vi "path steer3.vi"(11 "lane":bool) -> (2 "curve vel limit":dbl, 3 "handle":dbl=175.61695170488764)   [LabVIEW 2015]
uses:
  <vilib>/Analysis/7linalg.llb/Solve Linear Equations (single right hand).vi
  <vilib>/Analysis/baseanly.llb/Solve Linear Equations By Cholesky.vi
  <vilib>/Analysis/baseanly.llb/Real Matrix to Compact Array.vi
  <vilib>/Analysis/baseanly.llb/Real Compact Tri-Matrix Linear Eqs.vi
  G_ALL.vi
  <vilib>/Analysis/7linalg.llb/Solve Linear Eqs (General).vi
  <vilib>/Analysis/7linalg.llb/Solve Linear Eqs (Gen, single right hand).vi
  <vilib>/Analysis/NI_AALPro.lvlib
panel:
  out "path end":bool
  in  "an[g]":dbl=-0.17 format="%#_13g"
  out "Waveform Graph":dynamicdata(graph)
  in  "mu":dbl=0.005 format="%#_13g"
  in  "dx gain":dbl=0.019999999999999997 min=0.0 max=0.2 step=0.01
  out "x value":dbl=-0.8542483758567541
  out "XY Graph":cluster{"Y":dbl[], "Y":dbl[]}[](graph)=[{"Y"=[-5.246809304707959, -4.763210909809536, -4.298248751776158, -3.853163667485589, -3.4268765479315446, -3.029477672753705, -2.6673284986480974, -2.335336691519628, -2.0366453167866156, -1.7750835921098853, -1.5528767688369498, -1.3644656447475765, -1.2079630605299954, -1.074690008661569, -0.9585132340675446, -0.8551782329420596, -0.7665829934540727, -0.6868993462607671, -0.6126823280970868, -0.5442164343365972, -0.47614894814750475, -0.41410047141640827, -0.3538150238541624, -0.29540366128691464, -0.24219086500490516, -0.19691528446819184, -0.15547027846011519, -0.11340295527325328, -0.07144915398020535, -0.03434793001665748, 0.0, 0.026526158792223087, 0.05124494389382517, 0.07270742281515652, 0.06435385726912624, -0.004553363938687882, -0.139882839282637, -0.3359547912247316, -0.5900103181212502, -0.900040761768828, -1.2577413584671457, -1.66216965308078, -2.1012210225275174, -2.5653232377446606, -3.0450206197370466, -3.5404770109177743, -4.039369871326692, -4.541851143281866, -5.046387603513992, -5.553897537492966, -6.061637927692216, -6.567645563226444, -7.068648217182836, -7.570715384980373, -8.064438697718192, -8.545111556606587, -8.998477174205098, -9.422019565773061, -9.805695724849244, -10.146105279341642], "Y"=[-13.12635530502614, -12.964543503689939, -12.76763447744193, -12.524937360608902, -12.2475735581719, -11.933583222485607, -11.583671941038977, -11.206464906204559, -10.79245190322264, -10.354599285401152, -9.898639757724679, -9.426030687571156, -8.945680321385996, -8.454465203163156, -7.963985068856038, -7.468786738899853, -6.97312085053041, -6.479311060157665, -5.971731167568438, -5.469535412616666, -4.9636888467403155, -4.464752828537232, -3.9649913085777393, -3.458342585235778, -2.9601418499725303, -2.459972000641257, -1.9586644185731306, -1.4494467342092758, -0.9454480119816643, -0.4403687170997531, 0.06136222931732077, 0.5678735764406926, 1.068808881478275, 1.5686590067794068, 2.0720530905057277, 2.5736288544042853, 3.0594879994083963, 3.5248827445502124, 3.9579216058298154, 4.3560080630331335, 4.707794061133773, 5.011781058067703, 5.259264085768475, 5.451142759582283, 5.593309208559008, 5.693936293621469, 5.758617125078806, 5.791664966026638, 5.794000380643315, 5.784136801290129, 5.782533687658117, 5.785062966223215, 5.79993550563809, 5.8290421589798, 5.9156579447766475, 6.067163605595132, 6.278887512503447, 6.54911596168099, 6.871713294872911, 7.24413426029683]}, {"Y"=[-27.79054311036769, -27.788426793206575, -27.782078486373944, -27.77150012362555, -27.75669492723317, -27.737667407003034, -27.71442335890214, -27.686969863292695, -27.655315282775426, -27.619469259642194, -27.5794427129389, -27.5352478351394, -27.48689808843162, -27.434408200616765, -27.377794160623147, -27.317073213635787, -27.25226385584335, -27.18338582880404, -27.110460113432133, -27.033508923606977, -26.95255569940644, -26.867625099966816, -26.77874299597144, -26.68593646177021, -26.589233767132484, -26.488664368635824, -26.384258900693254, -26.2760491662217, -26.16406812695454, -26.048349893401117, -25.92892971445636, -25.805843966663623, -25.679130143134046, -25.548826842125777, -25.41497375528658, -25.27761165556337, -25.13678238478238, -24.992528840903734, -24.844894964954314, -24.693925727642892, -24.53966711566163, -24.382166117678068, -24.221470710021944, -24.057629842071115, -23.890693421341133, -23.720712298282884, -23.547738250793113, -23.37182396844231, -23.193023036425007, -23.011389919237175, -22.82697994408583, -22.639849284035826, -22.450054940898987, -22.257654727870808, -22.062707251920006, -21.865271895936253, -21.66540880064158, -21.463178846270928, -21.25864363402745, -21.05186546731817, -20.84290733277577, -20.631832881072256, -20.41870640753034, -20.20359283253847, -19.986557681775434, -19.767667066250628, -19.54698766216598, -19.324586690605734, -19.10053189706029, -18.874891530790215, -18.64773432403691, -18.419129471086073, -18.18914660719046, -17.957855787358298, -17.725327465013883, -17.491632470536747, -17.256841989686063, -17.02102754191677, -16.784260958594032, -16.546614361112756, -16.308160138928653, -16.068970927507767, -15.829119586200973, -15.588679176050324, -15.347722937533948, -15.106324268256303, -14.864556700590517, -14.622493879279771, -14.38020953900434, -14.137777481921338, -13.895271555183845, -13.652765628446353, -13.410333571363354, -13.16804923108792, -12.92598640977717, -12.684218842111388, -12.442820172833741, -12.20186393431737, -11.961423524166722, -11.721572182859921, -11.482382971439037, -11.243928749254936, -11.006282151773657, -10.769515568450924, -10.533701120681629, -10.298910639830943, -10.06521564535381, -9.832687323009392, -9.601396503177233, -9.37141363928162, -9.142808786330779, -8.915651579577474, -8.690011213307402, -8.465956419761957, -8.243555448201716, -8.022876044117066, -7.803985428592254, -7.586950277829223, -7.371836702837354, -7.158710229295436, -6.947635777591925, -6.738677643049522, -6.531899476340242, -6.32736426409676, -6.125134309726112, -5.925271214431441, -5.727835858447683, -5.53288838249688, -5.3404881694687045, -5.150693826331867, -4.96356316628186, -4.779153191130517, -4.597520073942688, -4.418719141925381, -4.242804859574576, -4.069830812084804, -3.8998496890265617, -3.7329132682965724, -3.5690724003457444, -3.4083769926896217, -3.250875994706062, -3.096617382724796, -2.9456481454133776, -2.798014269463957, -2.6537607255853093, -2.5129314548043187, -2.3755693550811117, -2.241716268241916, -2.1114129672336457, -1.9846991437040682, -1.8616133959113306, -1.7421932169665748, -1.62647498341315, -1.5144939441459915, -1.406284209674439, -1.3018787417318656, -1.201309343235204, -1.1046066485974766, -1.0118001143962498, -0.9229180104008776, -0.8379874109612526, -0.7570341867607127, -0.6800829969355568, -0.6071572815636515, -0.5382792545243404, -0.47346989673190265, -0.41274894974454135, -0.3561349097509261, -0.30364502193607024, -0.25529527522828666, -0.21110039742879394, -0.1710738507254952, -0.13522782759226182, -0.10357324707499238, -0.07611975146555316, -0.052875703364655635, -0.03384818313452165, -0.019042986742137558, -0.00846462399374559, -0.0021163171611142673, 0.0, -0.0021163171611142673, -0.00846462399374559, -0.019042986742137558, -0.03384818313452165, -0.052875703364655635, -0.07611975146555316, -0.10357324707499238, -0.13522782759226182, -0.17107385072549341, -0.21110039742879394, -0.25529527522828666, -0.30364502193607024, -0.3561349097509261, -0.4127489497445396, -0.4734698967319009, -0.5382792545243387, -0.6071572815636497, -0.6800829969355586, -0.7570341867607127, -0.8379874109612526, -0.9229180104008758, -1.011800114396248, -1.1046066485974766, -1.2013093432352022, -1.3018787417318638, -1.4062842096744355, -1.5144939441459861, -1.6264749834131482, -1.7421932169665766, -1.8616133959113323, -1.9846991437040664, -2.111412967233644, -2.2417162682419143, -2.37556935508111, -2.512931454804317, -2.6537607255853075, -2.798014269463952, -2.9456481454133705, -3.0966173827247943, -3.2508759947060604, -3.4083769926896235, -3.569072400345746, -3.7329132682965707, -3.89984968902656, -4.069830812084803, -4.242804859574575, -4.418719141925379, -4.597520073942681, -4.77915319113051, -4.9635631662818565, -5.150693826331869, -5.340488169468708, -5.532888382496882, -5.727835858447682, -5.925271214431433, -6.125134309726104, -6.3273642640967624, -6.531899476340239, -6.738677643049519, -6.947635777591917, -7.158710229295428, -7.371836702837351, -7.58695027782922, -7.803985428592251, -8.022876044117067, -8.243555448201715, -8.465956419761955, -8.6900112133074, -8.915651579577467, -9.14280878633077, -9.371413639281617, -9.601396503177229, -9.832687323009386, -10.065215645353812, -10.298910639830945, -10.533701120681625, -10.769515568450919, -11.006282151773648, -11.24392874925494, -11.482382971439037, -11.721572182859921, -11.961423524166714, -12.201863934317359, -12.442820172833729, -12.684218842111388, -12.925986409777169, -13.168049231087927, -13.410333571363354, -13.652765628446351, -13.895271555183843, -14.137777481921333, -14.380209539004332, -14.622493879279759, -14.864556700590516, -15.106324268256296, -15.347722937533955, -15.588679176050325, -15.82911958620097, -16.068970927507763, -16.30816013892865, -16.546614361112745, -16.784260958594036, -17.021027541916766, -17.25684198968606, -17.49163247053674, -17.725327465013873, -17.957855787358298, -18.189146607190455, -18.41912947108607, -18.647734324036914, -18.874891530790215, -19.100531897060286, -19.32458669060573, -19.546987662165968, -19.767667066250617, -19.986557681775434, -20.203592832538465, -20.418706407530333, -20.631832881072256, -20.842907332775766, -21.051865467318166, -21.258643634027447, -21.46317884627092, -21.66540880064158, -21.865271895936253, -22.062707251920003, -22.257654727870804, -22.45005494089898, -22.63984928403582, -22.826979944085828, -23.01138991923717, -23.19302303642501, -23.371823968442314, -23.54773825079311, -23.720712298282884, -23.890693421341126, -24.057629842071112, -24.221470710021936, -24.382166117678068, -24.539667115661626, -24.693925727642895, -24.844894964954314, -24.992528840903734, -25.13678238478238, -25.277611655563366, -25.414973755286574, -25.548826842125777, -25.679130143134046, -25.805843966663623, -25.928929714456356, -26.04834989340111, -26.16406812695454, -26.276049166221696, -26.384258900693247, -26.488664368635824, -26.589233767132484, -26.68593646177021, -26.778742995971438, -26.867625099966812, -26.95255569940643, -27.033508923606977, -27.110460113432133, -27.183385828804038, -27.25226385584335, -27.317073213635787, -27.377794160623147, -27.434408200616765, -27.486898088431616, -27.535247835139405, -27.5794427129389, -27.619469259642194, -27.655315282775426, -27.686969863292695, -27.71442335890214, -27.737667407003034, -27.75669492723317, -27.77150012362555, -27.782078486373944, -27.788426793206575], "Y"=[-0.0, -0.24250592673749302, -0.48493798382049413, -0.7272223240959237, -0.969285145406673, -1.2110527130724553, -1.4524513823501046, -1.6934076208664777, -1.9338480310171269, -2.1736993723239215, -2.4128885837448077, -2.6513428059289086, -2.8889894034101893, -3.1257559867329223, -3.3615704345022186, -3.596360915352901, -3.830055909830037, -4.062584232174453, -4.293875052006613, -4.52385791590223, -4.752462768853066, -4.97961997560637, -5.205260341876442, -5.429315135421889, -5.65171610698213, -5.872395511066782, -6.091286126591589, -6.308321277354623, -6.523434852346495, -6.736561325888409, -6.9476357775919215, -7.156593912134322, -7.363372078843605, -7.567907291087082, -7.770137245457733, -7.970000340752407, -8.167435696736161, -8.362383172686963, -8.55478338571514, -8.744577728851981, -8.931708388901985, -9.11611836405333, -9.29775148124116, -9.476552413258466, -9.652466695609267, -9.82544074309904, -9.995421866157285, -10.162358286887272, -10.326199154838099, -10.486894562494223, -10.644395560477784, -10.798654172459047, -10.949623409770469, -11.09725728571989, -11.241510829598536, -11.382340100379524, -11.519702200102733, -11.65355528694193, -11.783858587950201, -11.910572411479777, -12.033658159272512, -12.15307833821727, -12.268796571770693, -12.380777611037853, -12.488987345509406, -12.59339281345198, -12.693962211948639, -12.790664906586368, -12.883471440787595, -12.97235354478297, -13.057284144222592, -13.138237368423132, -13.215188558248288, -13.288114273620195, -13.356992300659504, -13.421801658451942, -13.482522605439303, -13.539136645432919, -13.591626533247775, -13.639976279955558, -13.684171157755053, -13.72419770445835, -13.760043727591583, -13.791698308108852, -13.819151803718292, -13.84239585181919, -13.861423372049323, -13.876228568441707, -13.8868069311901, -13.89315523802273, -13.895271555183845, -13.89315523802273, -13.8868069311901, -13.876228568441707, -13.861423372049323, -13.84239585181919, -13.819151803718293, -13.791698308108852, -13.760043727591583, -13.72419770445835, -13.684171157755053, -13.639976279955558, -13.591626533247775, -13.53913664543292, -13.482522605439303, -13.421801658451942, -13.356992300659504, -13.288114273620195, -13.215188558248288, -13.138237368423134, -13.057284144222592, -12.972353544782969, -12.883471440787595, -12.790664906586368, -12.69396221194864, -12.593392813451981, -12.488987345509406, -12.380777611037855, -12.268796571770697, -12.153078338217272, -12.033658159272516, -11.910572411479778, -11.783858587950201, -11.65355528694193, -11.519702200102735, -11.382340100379528, -11.241510829598536, -11.09725728571989, -10.949623409770469, -10.79865417245905, -10.644395560477784, -10.486894562494225, -10.326199154838102, -10.162358286887274, -9.995421866157285, -9.825440743099042, -9.65246669560927, -9.476552413258466, -9.297751481241159, -9.11611836405333, -8.931708388901988, -8.74457772885198, -8.554783385715142, -8.362383172686968, -8.167435696736163, -7.9700003407524065, -7.770137245457734, -7.567907291087087, -7.363372078843605, -7.1565939121343245, -6.9476357775919215, -6.7365613258884105, -6.523434852346494, -6.308321277354625, -6.091286126591593, -5.872395511066783, -5.6517161069821285, -5.42931513542189, -5.205260341876445, -4.979619975606376, -4.752462768853069, -4.523857915902228, -4.293875052006615, -4.062584232174458, -3.8300559098300377, -3.596360915352905, -3.361570434502219, -3.1257559867329254, -2.888989403410189, -2.6513428059289113, -2.4128885837448126, -2.1736993723239233, -1.933848031017125, -1.6934076208664786, -1.4524513823501084, -1.2110527130724555, -0.969285145406676, -0.7272223240959296, -0.4849379838204965, -0.24250592673749197, -1.7016237834565482e-15, 0.24250592673748858, 0.4849379838204931, 0.72722232409592, 0.9692851454066664, 1.2110527130724522, 1.4524513823501048, 1.6934076208664814, 1.9338480310171278, 2.1736993723239197, 2.4128885837448095, 2.6513428059289077, 2.8889894034101857, 3.1257559867329223, 3.3615704345022155, 3.5963609153528955, 3.830055909830029, 4.062584232174455, 4.293875052006618, 4.523857915902231, 4.752462768853065, 4.979619975606372, 5.205260341876442, 5.429315135421887, 5.651716106982125, 5.872395511066779, 6.0912861265915845, 6.308321277354616, 6.52343485234649, 6.736561325888413, 6.947635777591924, 7.156593912134322, 7.363372078843602, 7.567907291087084, 7.7701372454577315, 7.970000340752404, 8.16743569673616, 8.36238317268696, 8.554783385715135, 8.744577728851977, 8.931708388901985, 9.116118364053332, 9.29775148124116, 9.476552413258464, 9.652466695609267, 9.825440743099039, 9.995421866157281, 10.162358286887272, 10.326199154838095, 10.48689456249422, 10.644395560477783, 10.798654172459052, 10.94962340977047, 11.09725728571989, 11.241510829598534, 11.382340100379523, 11.51970220010273, 11.653555286941932, 11.7838585879502, 11.910572411479777, 12.03365815927251, 12.153078338217266, 12.268796571770695, 12.380777611037853, 12.488987345509404, 12.593392813451981, 12.69396221194864, 12.790664906586366, 12.883471440787595, 12.972353544782967, 13.057284144222589, 13.138237368423132, 13.215188558248288, 13.288114273620193, 13.356992300659506, 13.421801658451942, 13.482522605439303, 13.539136645432919, 13.591626533247773, 13.63997627995556, 13.684171157755053, 13.72419770445835, 13.760043727591581, 13.791698308108852, 13.819151803718292, 13.84239585181919, 13.861423372049323, 13.876228568441707, 13.8868069311901, 13.89315523802273, 13.895271555183845, 13.89315523802273, 13.8868069311901, 13.876228568441707, 13.861423372049323, 13.84239585181919, 13.819151803718292, 13.791698308108852, 13.760043727591583, 13.724197704458351, 13.684171157755053, 13.63997627995556, 13.591626533247773, 13.539136645432919, 13.482522605439305, 13.421801658451944, 13.356992300659506, 13.288114273620195, 13.21518855824829, 13.138237368423134, 13.05728414422259, 12.972353544782969, 12.883471440787597, 12.79066490658637, 12.693962211948643, 12.593392813451985, 12.488987345509408, 12.380777611037855, 12.268796571770697, 12.15307833821727, 12.033658159272512, 11.910572411479778, 11.783858587950203, 11.653555286941934, 11.519702200102733, 11.382340100379524, 11.241510829598537, 11.097257285719893, 10.949623409770474, 10.798654172459056, 10.644395560477784, 10.486894562494227, 10.326199154838095, 10.16235828688727, 9.995421866157285, 9.825440743099042, 9.65246669560927, 9.47655241325847, 9.29775148124117, 9.11611836405333, 8.931708388901988, 8.744577728851976, 8.554783385715139, 8.362383172686963, 8.167435696736165, 7.970000340752413, 7.770137245457741, 7.567907291087083, 7.363372078843606, 7.156593912134326, 6.947635777591929, 6.736561325888418, 6.523434852346495, 6.308321277354626, 6.091286126591594, 5.872395511066778, 5.65171610698213, 5.429315135421891, 5.205260341876446, 4.979619975606377, 4.752462768853076, 4.52385791590223, 4.293875052006616, 4.062584232174459, 3.8300559098300337, 3.5963609153529004, 3.3615704345022204, 3.125755986732927, 2.888989403410197, 2.651342805928907, 2.4128885837448086, 2.173699372323925, 1.9338480310171329, 1.6934076208664863, 1.4524513823501162, 1.2110527130724573, 0.9692851454066778, 0.7272223240959189, 0.484937983820492, 0.24250592673749366]}]
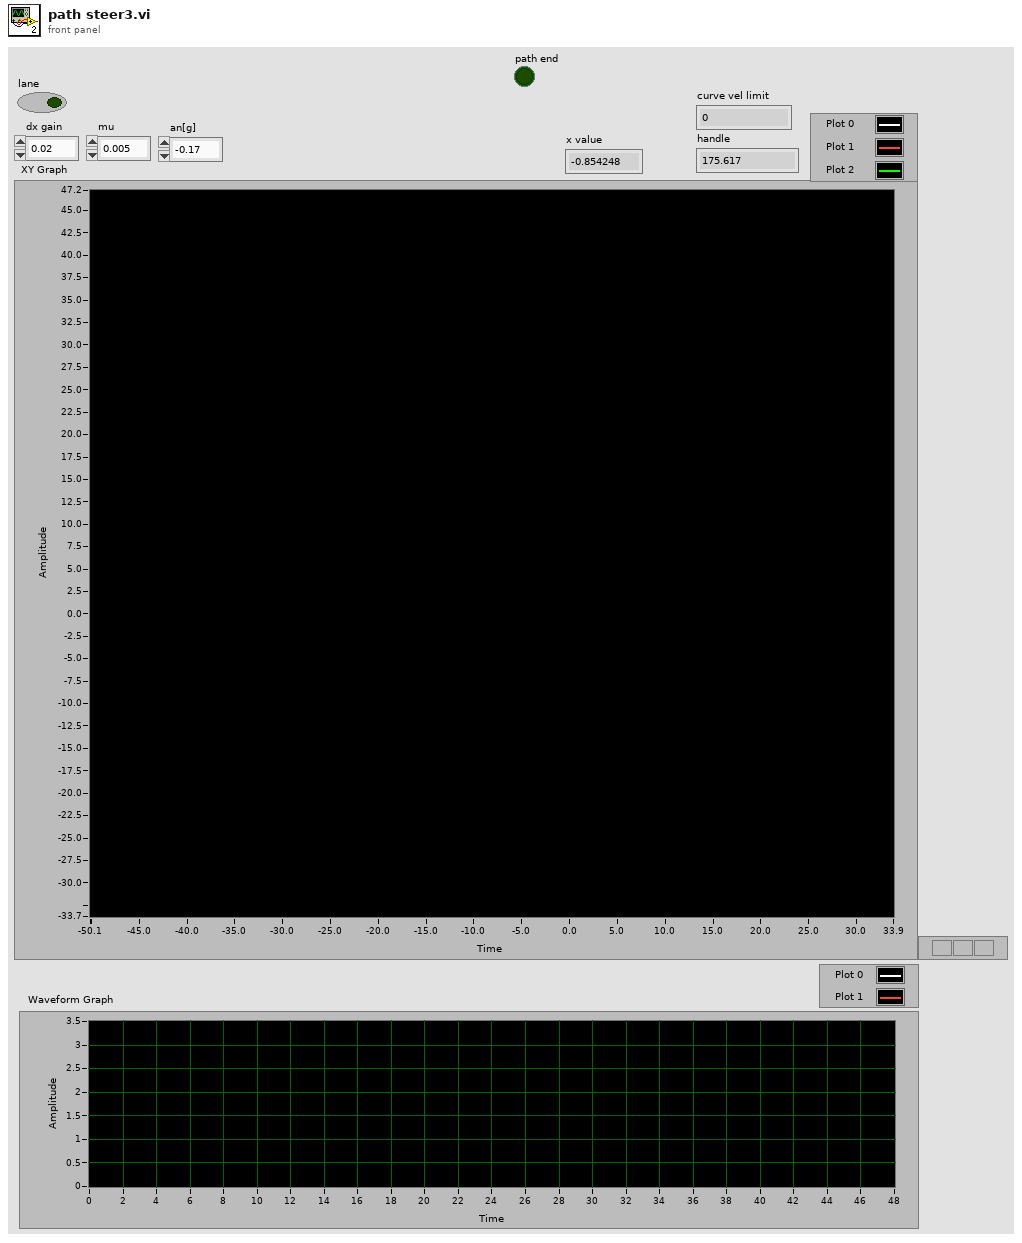
[diagram p1: front panel]
types:
  T1 = cluster{"Steer_input":dbl, "Steer_output":dbl, "VS_des":dbl, "VS_can":dbl, "heading":dbl, "auto":bool, "run":bool, "x":dbl, "y":dbl}
  T2 = cluster{"C_Wheel base":dbl, "ratio_steer":dbl, "Overall width":dbl, "af":dbl, "turn radius":dbl, "eval":dbl, "ap":dbl, "an":dbl, "Vmax":dbl, "mu":dbl, "Vlast":dbl}
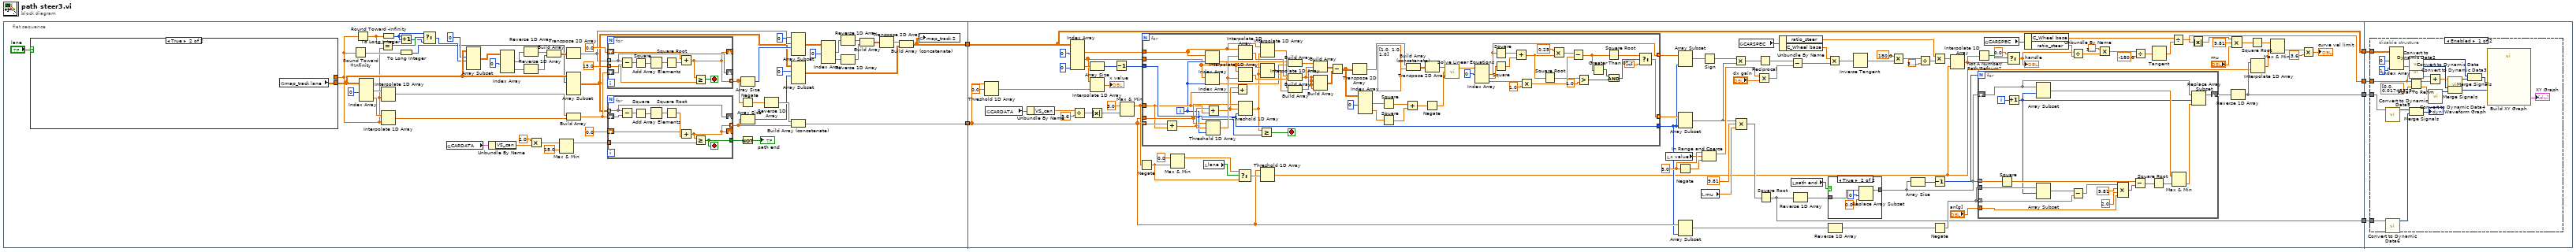
[diagram p0: block diagram]
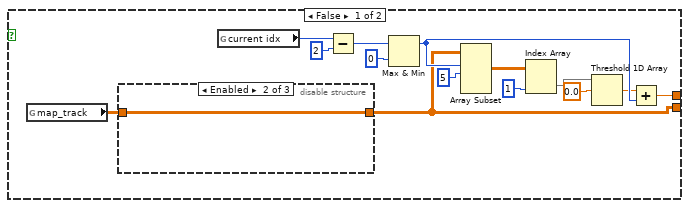
[diagram p2: hidden frame]
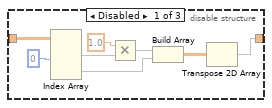
[diagram p3: hidden frame]
diagram:
  n1 = flat-sequence {
    tunnel: [w15] -> w5
    tunnel: [w14] -> w3
    tunnel: [w132] -> w6
    tunnel: w5 -> [w168]
    tunnel: [w168] -> w4
    tunnel: w3 -> [w124]
    tunnel: [w116] -> w2
    tunnel: [w115] -> w1
    tunnel: w6 -> [w276]
    tunnel: w4 -> [w277]
    tunnel: w2 -> [w275]
    tunnel: w1 -> [w274]
    frame #0 {
      n2 = case shown="True" "lane" {
        tunnel: [w63 w86] -> w53
        tunnel: [w65 _] -> w16
        frame False {
          n3 = global read "G_ALL.vi" "map_track"() -> (w64:dbl[][])
          n4 = disable-structure shown="Enabled" {
            disable-tunnel: w64 -> [w84 w85 _]
            disable-tunnel: [w77 w85 _] -> w63
            frame Disabled {
              n5 = Index Array(array=w84, index (col) #1=0 ("disabled index (col)")) -> (element #1=w82:dbl[], element #2=w79:dbl[])  [unwired: 3 in]
              n6 = Multiply(x=1.0, y=w82) -> (x*y=w80:dbl[])
              n7 = Build Array(w80, w79) -> (w78:dbl[][])
              n8 = Transpose 2D Array(2D array=w78) -> (transposed array=w77:dbl[][])
            }
            frame Enabled {
            }
            frame Disabled {
            }
          }
          n9 = global read "G_ALL.vi" "current idx"() -> (w66:i32)
          n10 = Subtract(x=w66, y=2) -> (x-y=w75:i32)
          n11 = Max & Min(x=w75, y=0) -> (max(x,y)=w69:i32)  [unwired: 1 out]
          n12 = Array Subset(array=w63, index (row)=w69, length (row)=5 ("length")) -> (w72:dbl[][])  [unwired: 2 in]
          n13 = Index Array(array=w72, index (col)=1 ("disabled index (col)")) -> (element=w70:dbl[])  [unwired: 1 in]
          n14 = Threshold 1D Array(2:0.0 ("threshold y"), 3:w70) -> (0:w67:dbl)  [unwired: 1 in]
          n15 = Add(x=w67, y=w69) -> (x+y=w65:dbl)
        }
        frame True {
          n16 = global read "G_ALL.vi" "map_track lane"() -> (w86:dbl[][])
        }
      }
      n17 = Round Toward +Infinity(x=w16) -> (ceil(x): smallest int >= x=w24:dbl)
      n18 = Round Toward -Infinity(1:w16) -> (0:w23:dbl)
      n19 = Index Array(array=w53, index (col) #1=0 ("disabled index (col)")) -> (element #1=w61:dbl[], element #2=w60:dbl[])  [unwired: 3 in]
      n20 = Equal?(x=w23, y=w16) -> (x = y?=w22:bool)
      n21 = To Long Integer(number=w23) -> (32bit integer=w20:i32)
      n22 = Interpolate 1D Array(1:w16, 2:w61) -> (0:w59:dbl)
      n23 = Interpolate 1D Array(1:w16, 2:w60) -> (0:w58:dbl)
      n24 = Increment(x=w20) -> (x+1=w19:i32)
      n25 = To Long Integer(number=w24) -> (32bit integer=w18:i32)
      n26 = Select(t=w20, s=w22, f=w19) -> (s? t:f=w21:i32)
      n27 = global read "G_ALL.vi" "CARDATA"() -> (w55:T1)
      n28 = Array Subset(array=w53, index (row)=0 ("index"), length (row)=w21) -> (w51:dbl[][])  [unwired: 2 in]
      n29 = Unbundle By Name(w55) -> ("VS_can"=w13:dbl)
      n30 = Index Array(array=w51, index (col) #1=0 ("disabled index (col)")) -> (element #1=w49:dbl[], element #2=w48:dbl[])  [unwired: 3 in]
      n31 = Reverse 1D Array(array=w49) -> (reversed array=w47:dbl[])
      n32 = Reverse 1D Array(array=w48) -> (reversed array=w46:dbl[])
      n33 = Multiply(x=2.0, y=w13) -> (x*y=w12:dbl)
      n34 = Build Array(w47, w46) -> (w26:dbl[][])
      n35 = Max & Min(x=w12, y=15.0) -> (max(x,y)=w54:dbl)  [unwired: 1 out]
      n36 = Transpose 2D Array(2D array=w26) -> (transposed array=w25:dbl[][])
      n37 = Array Subset(array=w53, index (row)=w18) -> (w28:dbl[][])  [unwired: 3 in]
      n38 = Build Array(w59, w58) -> (w44:dbl[])
      n39 = for {
        tunnel: w25 -> [w89] mode=indexing
        shift-right: [w89] -> _
        shift-left: w44 -> [w96]
        shift-right: [w88] -> _
        shift-left: 0.0 -> [w91]
        tunnel: 15.0 ("y") -> [w90]
        tunnel: [w88] -> w40 mode=indexing
        stop <- w87 stop-if-true
        n40 = Subtract(x=w89, y=w96) -> (x-y=w95:dbl[])
        n41 = Square(x=w95) -> (x^2=w94:dbl[])
        n42 = Add Array Elements(numeric array=w94) -> (sum=w93:dbl)
        n43 = Square Root(x=w93) -> (sqrt(x)=w92:dbl)
        n44 = Add(x=w91, y=w92) -> (x+y=w88:dbl)
        n45 = Greater Or Equal?(x=w88, y=w90) -> (x >= y?=w87:bool)
      }
      n46 = for {
        tunnel: w28 -> [w99] mode=indexing
        shift-right: [w99] -> _
        shift-left: w44 -> [w106]
        shift-right: [w98] -> _
        shift-left: 0.0 -> [w101]
        tunnel: w54 -> [w100]
        tunnel: [w98] -> w27 mode=indexing
        tunnel: [w97] -> w8
        stop <- w97 stop-if-true
        n47 = Subtract(x=w99, y=w106) -> (x-y=w105:dbl[])
        n48 = Square(x=w105) -> (x^2=w104:dbl[])
        n49 = Add Array Elements(numeric array=w104) -> (sum=w103:dbl)
        n50 = Square Root(x=w103) -> (sqrt(x)=w102:dbl)
        n51 = Add(x=w101, y=w102) -> (x+y=w98:dbl)
        n52 = Greater Or Equal?(x=w98, y=w100) -> (x >= y?=w97:bool)
      }
      n53 = Negate(x=w40) -> (-x=w42:dbl[])
      n54 = Not(x=w8) -> (.not. x?=→"path end":bool)
      n55 = Array Size(array=w40) -> (size(s)=w38:i32)
      n56 = Array Size(array=w27) -> (size(s)=w9:i32)
      n57 = Reverse 1D Array(array=w42) -> (reversed array=w41:dbl[])
      n58 = Array Subset(array=w25, index (row)=0 ("index"), length (row)=w38) -> (w33:dbl[][])  [unwired: 2 in]
      n59 = Array Subset(array=w28, index (row)=0 ("index"), length (row)=w9) -> (w10:dbl[][])  [unwired: 2 in]
      n60 = Build Array (concatenate)(w41, w27) -> (w14:dbl[])
      n61 = Index Array(array=w33, index (col) #1=0 ("disabled index (col)")) -> (element #1=w32:dbl[], element #2=w31:dbl[])  [unwired: 3 in]
      n62 = Reverse 1D Array(array=w32) -> (reversed array=w35:dbl[])
      n63 = Reverse 1D Array(array=w31) -> (reversed array=w36:dbl[])
      n64 = Build Array(w35, w36) -> (w37:dbl[][])
      n65 = Transpose 2D Array(2D array=w37) -> (transposed array=w30:dbl[][])
      n66 = Build Array (concatenate)(w30, w10) -> (w15:dbl[][])
      n67 = global write "G_ALL.vi" "map_track 2"(w15) -> ()
    }
    frame #1 {
      w147 = 5.0 ("upper limit")
      n68 = Threshold 1D Array(2:0.0 ("threshold y"), 3:w124) -> (0:w173:dbl)  [unwired: 1 in]
      n69 = global read "G_ALL.vi" "CARDATA"() -> (w167:T1)
      n70 = Unbundle By Name(w167) -> ("VS_can"=w166:dbl)
      n71 = Index Array(array=w168, index (col) #1=0 ("disabled index (col)"), index (col) #3=0 ("index (col)")) -> (element #1=w193:dbl[], element #2=w172:dbl[], element #3=w170:dbl[])  [unwired: 4 in]
      n72 = Divide(x=w166, y=3.6) -> (x/y=w155:dbl)
      n73 = Absolute Value(x=w155) -> (abs(x)=w154:dbl)
      n74 = Array Size(array=w172) -> (size(s)=w192:i32)
      n75 = Interpolate 1D Array(1:w173, 2:w170) -> (0:→"x value":dbl)
      n76 = Decrement(x=w192) -> (x-1=w191:i32)
      n77 = Max & Min(x=3.0, y=w154) -> (max(x,y)=w152:dbl)  [unwired: 1 out]
      n78 = Negate(x=w152) -> (-x=w140:dbl)
      n79 = for {
        tunnel: w124 -> [w225]
        tunnel: w124 -> [w273] mode=indexing
        tunnel: w193 -> [w221]
        tunnel: w172 -> [w220]
        tunnel: [w239] -> w190 mode=indexing
        tunnel: w191 -> [w238]
        tunnel: [w236] -> w189 mode=indexing
        tunnel: [w222] -> w123
        tunnel: w152 -> [w223]
        i -> [w222]
        stop <- w237 stop-if-true
        n80 = Add(x=w273, y=w223) -> (x+y=w269:dbl)
        n81 = Index Array(array=w221, index=w222) -> (element=w265:dbl)
        n82 = Index Array(array=w220, index=w222) -> (element=w264:dbl)
        n83 = Threshold 1D Array(1:w222, 2:w269, 3:w225) -> (0:w272:dbl)
        n84 = Add(x=w269, y=w223) -> (x+y=w224:dbl)
        n85 = Add(x=w224, y=w223) -> ()  [unwired: 1 out]
        n86 = Interpolate 1D Array(1:w272, 2:w221) -> (0:w270:dbl)
        n87 = Interpolate 1D Array(1:w272, 2:w220) -> (0:w271:dbl)
        n88 = Threshold 1D Array(1:w222, 2:w224, 3:w225) -> (0:w218:dbl)
        n89 = Greater Or Equal?(x=w218, y=w238) -> (x >= y?=w237:bool)
        n90 = Interpolate 1D Array(1:w218, 2:w221) -> (0:w268:dbl)
        n91 = Interpolate 1D Array(1:w218, 2:w220) -> (0:w267:dbl)
        n92 = Build Array(w265, w264) -> (w232:dbl[])
        n93 = Build Array(w270, w271) -> (w219:dbl[])
        n94 = Build Array(w268, w267) -> (w266:dbl[])
        n95 = Build Array(w232, w219, w266) -> (w235:dbl[][])
        n96 = Build Array(w219, w219, w219, w219) -> (w234:dbl[][])
        n97 = Subtract(x=w235, y=w234) -> (x-y=w233:dbl[][])
        n98 = Transpose 2D Array(2D array=w233) -> (transposed array=w245:dbl[][])
        n99 = Index Array(array=w233, index (col) #1=0 ("disabled index (col)")) -> (element #1=w241:dbl[], element #2=w242:dbl[])  [unwired: 3 in]
        n100 = Square(x=w241) -> (x^2=w243:dbl[])
        n101 = Square(x=w242) -> (x^2=w244:dbl[])
        n102 = Add(x=w243, y=w244) -> (x+y=w246:dbl[])
        n103 = Build Array (concatenate)(w245, dbl[] [1.0, 1.0, 1.0] ("initialized array")) -> (w255:dbl[][])
        n104 = Negate(x=w246) -> (-x=w247:dbl[])
        n105 = Transpose 2D Array(2D array=w255) -> (transposed array=w256:dbl[][])
        n106 = call-poly <vilib>:"Solve Linear Equations.vi"("Known Vector"=w247, "Input Matrix"=w256) -> ("Solution Vector"=w248:dbl[])  [unwired: 1 in, 1 out]
        n107 = Index Array(array=w248, index #1=0 ("index")) -> (element #1=w236:dbl, element #2=w250:dbl, element #3=w253:dbl)  [unwired: 2 in]
        n108 = Square(x=w236) -> (x^2=w251:dbl)
        n109 = Square(x=w250) -> (x^2=w252:dbl)
        n110 = Add(x=w251, y=w252) -> (x+y=w231:dbl)
        n111 = Multiply(x=w253, y=1.0) -> (x*y=w254:dbl)
        n112 = Square Root(x=w231) -> (sqrt(x)=w230:dbl)
        n113 = Multiply(x=0.25, y=w231) -> (x*y=w261:dbl)
        n114 = Subtract(x=w261, y=w254) -> (x-y=w257:dbl)
        n115 = Greater?(x=w230, y=1.0) -> (0:w227:bool)
        n116 = Greater Than 0?(x=w257) -> (x > 0?=w228:bool)
        n117 = Square Root(x=w257) -> (sqrt(x)=w263:dbl)
        n118 = And(x=w228, y=w227) -> (x .and. y?=w226:bool)
        n119 = Select(t=w263, s=w226, f=inf) -> (s? t:f=w239:dbl)
      }
      n120 = Max & Min(x=0.0 ("t"), y=w140) -> (max(x,y)=w139:dbl)  [unwired: 1 out]
      n121 = local read "lane"() -> (w138:bool)
      n122 = Select(t=w139, s=w138, f=w140) -> (s? t:f=w151:dbl)
      n123 = Threshold 1D Array(2:w151, 3:w124) -> (0:w113:dbl)  [unwired: 1 in]
      n124 = local read "x value"() -> (w143:dbl)
      n125 = Negate(x=w147) -> (-x=w146:dbl)
      n126 = Array Subset(array=w189, length=w123) -> (w188:dbl[])  [unwired: 1 in]
      n127 = Array Subset(array=w190, length=w123) -> (w127:dbl[])  [unwired: 1 in]
      n128 = Array Subset(array=w124, length=w123) -> (w112:dbl[])  [unwired: 1 in]
      n129 = local read "mu"() -> (w128:dbl)
      n130 = In Range and Coerce(upper limit=w147, x=w143, lower limit=w146) -> (coerced(x)=w145:dbl)  [unwired: 1 out]
      n131 = Sign(1:w188) -> (0:w175:dbl[])
      n132 = Multiply(x=w175, y=w127) -> (x*y=w126:dbl[])
      n133 = Compound Arithmetic op=MULTIPLY(w127, 9.81 ("value"), w128) -> (w130:dbl[])
      n134 = global read "G_ALL.vi" "CARSPEC"() -> (w181:T2)
      n135 = Multiply(x=w145, y="dx gain") -> (x*y=w142:dbl)
      n136 = Reciprocal(x=w126) -> (1/x=w125:dbl[])
      n137 = Square Root(x=w130) -> (sqrt(x)=w115:dbl[])
      n138 = Unbundle By Name(w181) -> ("ratio_steer"=w179:dbl, "C_Wheel base"=w180:dbl)
      n139 = Subtract(x=w125, y=w142) -> (x-y=w149:dbl[])
      n140 = local read "path end"() -> (w109:bool)
      n141 = Reverse 1D Array(array=w115) -> (reversed array=w108:dbl[])
      n142 = Multiply(x=w180, y=w149) -> (x*y=w187:dbl[])
      n143 = case shown="True" w109 {
        tunnel: w108 -> [w195 w199]
        tunnel: [w195 w198] -> w107
        frame False {
        }
        frame True {
          n144 = Replace Array Subset(array=w199, new element=0.0 ("new element/subarray"), index=0) -> (w198:dbl[])
        }
      }
      n145 = Reverse 1D Array(array=w112) -> (reversed array=w122:dbl[])
      n146 = Inverse Tangent(1:w187) -> (0:w185:dbl[])
      n147 = Multiply(x=180.0 ("y"), y=w185) -> (x*y=w184:dbl[])
      n148 = Array Size(array=w107) -> (size(s)=w114:i32)
      n149 = Divide(x=w184, y=3.141592653589793) -> (x/y=w182:dbl[])
      n150 = Multiply(x=w179, y=w182) -> (x*y=w148:dbl[])
      n151 = Decrement(x=w114) -> (x-1=w120:i32)
      n152 = Negate(x=w122) -> (-x=w121:dbl[])
      n153 = Interpolate 1D Array(1:w113, 2:w148) -> (0:w176:dbl)
      n154 = Not A Number/Path/Refnum?(number/path/refnum=w176) -> (NaN/Path/Refnum?=w178:bool)
      n155 = for {
        N: w120 -> [_]
        tunnel: w107 -> [w215] mode=indexing
        tunnel: w121 -> [w216]
        shift-right: [w206] -> w117
        shift-left: w107 -> [w209]
        tunnel: w121 -> [w203] mode=indexing
        tunnel: "an[g]" -> [w200]
        i -> [w217]
        n156 = Square(x=w215) -> (x^2=w214:dbl)
        n157 = Increment(x=w217) -> (x+1=w208:i32)
        n158 = Array Subset(array=w209, index=w208) -> (w210:dbl[])  [unwired: 1 in]
        n159 = Array Subset(array=w216, index=w208) -> (w204:dbl[])  [unwired: 1 in]
        n160 = Subtract(x=w204, y=w203) -> (x-y=w202:dbl[])
        n161 = Compound Arithmetic op=MULTIPLY(w202, 9.81 ("value"), 2.0 ("value"), w200) -> (w212:dbl[])
        n162 = Subtract(x=w214, y=w212) -> (x-y=w211:dbl[])
        n163 = Square Root(x=w211) -> (sqrt(x)=w205:dbl[])
        n164 = Max & Min(x=w210, y=w205) -> (min(x,y)=w207:dbl[])  [unwired: 1 out]
        n165 = Replace Array Subset(array=w209, new element=w207, index=w208) -> (w206:dbl[])
      }
      n166 = global read "G_ALL.vi" "CARSPEC"() -> (w164:T2)
      n167 = Select(t=0.0, s=w178, f=w176) -> (s? t:f=w150:dbl)
      "handle" <- w150
      n168 = Unbundle By Name(w164) -> ("C_Wheel base"=w156:dbl, "ratio_steer"=w163:dbl)
      n169 = Divide(x=w150, y=w163) -> (x/y=w161:dbl)
      n170 = Multiply(x=3.141592653589793, y=w161) -> (x*y=w160:dbl)
      n171 = Divide(x=w160, y=-180.0) -> (x/y=w158:dbl)
      n172 = Tangent(1:w158) -> (0:w157:dbl)
      n173 = Divide(x=w156, y=w157) -> (x/y=w132:dbl)
      n174 = Absolute Value(x=w132) -> (abs(x)=w131:dbl)
      n175 = Reverse 1D Array(array=w117) -> (reversed array=w116:dbl[])
      n176 = Compound Arithmetic op=MULTIPLY(w131, 9.81 ("value"), "mu") -> (w135:dbl)
      n177 = Square Root(x=w135) -> (sqrt(x)=w119:dbl)
      n178 = Interpolate 1D Array(1:w113, 2:w116) -> (0:w118:dbl)
      n179 = Max & Min(x=w119, y=w118) -> (min(x,y)=w110:dbl)  [unwired: 1 out]
      n180 = Multiply(x=w110, y=3.6) -> (x*y=→"curve vel limit":dbl)
    }
    frame #2 {
      n181 = disable-structure shown="Enabled" {
        disable-tunnel: w276 -> [w285 _]
        disable-tunnel: w277 -> [w284 _]
        disable-tunnel: w275 -> [w280 _]
        disable-tunnel: w274 -> [w278 _]
        frame Enabled {
          n182 = call "Convert to Dynamic Data5"("Array"=w280) -> ("Dynamic Data Type"=w281:dynamicdata)  [unwired: 3 in]
          n183 = call "Convert to Dynamic Data6"("Array"=w278) -> ("Dynamic Data Type"=w279:dynamicdata)  [unwired: 3 in]
          n184 = Index Array(array=w284, index (col) #1=0 ("disabled index (col)"), index (col) #2=1 ("disabled index (col)")) -> (element #1=w283:dbl[], element #2=w286:dbl[])  [unwired: 2 in]
          n185 = call "Convert to Dynamic Data"("Array"=w283) -> ("Dynamic Data Type"=w296:dynamicdata)  [unwired: 3 in]
          n186 = call "Convert to Dynamic Data2"("Array"=w286) -> ("Dynamic Data Type"=w295:dynamicdata)  [unwired: 3 in]
          n187 = Polar To Re/Im(2:dbl[] [0.0, 0.017453292519943295, 0.03490658503988659, 0.05235987755982988, 0.06981317007977318, 0.08726646259971647, 0.10471975511965977, 0.12217304763960307, 0.13962634015954636, 0.15707963267948966, 0.17453292519943295, 0.19198621771937624, 0.20943951023931953, 0.22689280275926282, 0.24434609527920614, 0.2617993877991494, 0.2792526803190927, 0.296705972839036, 0.3141592653589793, 0.33161255787892263, 0.3490658503988659, 0.3665191429188092, 0.3839724354387525, 0.40142572795869574, 0.41887902047863906, 0.4363323129985824, 0.45378560551852565, 0.47123889803846897, 0.4886921905584123, 0.5061454830783556, 0.5235987755982988, 0.5410520681182421, 0.5585053606381855, 0.5759586531581287, 0.593411945678072, 0.6108652381980153, 0.6283185307179586, 0.6457718232379019, 0.6632251157578453, 0.6806784082777886, 0.6981317007977318, 0.7155849933176751, 0.7330382858376184, 0.7504915783575618, 0.767944870877505, 0.7853981633974483, 0.8028514559173915, 0.8203047484373349, 0.8377580409572781, 0.8552113334772213, 0.8726646259971648, 0.890117918517108, 0.9075712110370513, 0.9250245035569946, 0.9424777960769379, 0.9599310885968813, 0.9773843811168246, 0.9948376736367678, 1.0122909661567112, 1.0297442586766543, 1.0471975511965976, 1.064650843716541, 1.0821041362364843, 1.0995574287564276, 1.117010721276371, 1.1344640137963142, 1.1519173063162573, 1.1693705988362009, 1.186823891356144, 1.2042771838760875, 1.2217304763960306, 1.239183768915974, 1.2566370614359172, 1.2740903539558606, 1.2915436464758039, 1.3089969389957472, 1.3264502315156905, 1.3439035240356336, 1.3613568165555772, 1.3788101090755203, 1.3962634015954636, 1.413716694115407, 1.4311699866353502, 1.4486232791552935, 1.4660765716752369, 1.48352986419518, 1.5009831567151235, 1.5184364492350666, 1.53588974175501, 1.5533430342749532, 1.5707963267948966, 1.5882496193148399, 1.605702911834783, 1.6231562043547265, 1.6406094968746698, 1.6580627893946132, 1.6755160819145563, 1.6929693744344996, 1.7104226669544427, 1.7278759594743864, 1.7453292519943295, 1.7627825445142729, 1.780235837034216, 1.7976891295541593, 1.8151424220741026, 1.8325957145940461, 1.8500490071139892, 1.8675022996339325, 1.8849555921538759, 1.902408884673819, 1.9198621771937625, 1.9373154697137058, 1.9547687622336491, 1.9722220547535922, 1.9896753472735356, 2.007128639793479, 2.0245819323134224, 2.0420352248333655, 2.0594885173533086, 2.076941809873252, 2.0943951023931953, 2.111848394913139, 2.129301687433082, 2.1467549799530254, 2.1642082724729685, 2.1816615649929116, 2.199114857512855, 2.2165681500327987, 2.234021442552742, 2.251474735072685, 2.2689280275926285, 2.2863813201125716, 2.3038346126325147, 2.321287905152458, 2.3387411976724017, 2.356194490192345, 2.373647782712288, 2.3911010752322315, 2.408554367752175, 2.426007660272118, 2.443460952792061, 2.4609142453120048, 2.478367537831948, 2.495820830351891, 2.5132741228718345, 2.530727415391778, 2.548180707911721, 2.5656340004316642, 2.5830872929516078, 2.600540585471551, 2.6179938779914944, 2.6354471705114375, 2.652900463031381, 2.670353755551324, 2.6878070480712672, 2.705260340591211, 2.7227136331111543, 2.7401669256310974, 2.7576202181510405, 2.7750735106709836, 2.792526803190927, 2.8099800957108707, 2.827433388230814, 2.844886680750757, 2.8623399732707004, 2.8797932657906435, 2.897246558310587, 2.91469985083053, 2.9321531433504737, 2.949606435870417, 2.96705972839036, 2.9845130209103035, 3.001966313430247, 3.01941960595019, 3.036872898470133, 3.0543261909900767, 3.07177948351002, 3.089232776029963, 3.1066860685499065, 3.12413936106985, 3.141592653589793, 3.159045946109736, 3.1764992386296798, 3.193952531149623, 3.211405823669566, 3.2288591161895095, 3.246312408709453, 3.2637657012293966, 3.2812189937493397, 3.2986722862692828, 3.3161255787892263, 3.3335788713091694, 3.3510321638291125, 3.368485456349056, 3.385938748868999, 3.4033920413889422, 3.4208453339088853, 3.4382986264288293, 3.455751918948773, 3.473205211468716, 3.490658503988659, 3.5081117965086026, 3.5255650890285457, 3.543018381548489, 3.560471674068432, 3.5779249665883754, 3.5953782591083185, 3.6128315516282616, 3.630284844148205, 3.647738136668149, 3.6651914291880923, 3.6826447217080354, 3.7000980142279785, 3.717551306747922, 3.735004599267865, 3.752457891787808, 3.7699111843077517, 3.787364476827695, 3.804817769347638, 3.8222710618675815, 3.839724354387525, 3.8571776469074686, 3.8746309394274117, 3.8920842319473548, 3.9095375244672983, 3.9269908169872414, 3.9444441095071845, 3.961897402027128, 3.979350694547071, 3.9968039870670142, 4.014257279586958, 4.031710572106902, 4.049163864626845, 4.066617157146788, 4.084070449666731, 4.101523742186674, 4.118977034706617, 4.136430327226561, 4.153883619746504, 4.171336912266447, 4.1887902047863905, 4.206243497306334, 4.223696789826278, 4.241150082346221, 4.258603374866164, 4.276056667386108, 4.293509959906051, 4.310963252425994, 4.328416544945937, 4.34586983746588, 4.363323129985823, 4.380776422505767, 4.39822971502571, 4.4156830075456535, 4.4331363000655974, 4.4505895925855405, 4.468042885105484, 4.485496177625427, 4.50294947014537, 4.520402762665314, 4.537856055185257, 4.5553093477052, 4.572762640225143, 4.590215932745086, 4.607669225265029, 4.625122517784973, 4.642575810304916, 4.66002910282486, 4.6774823953448035, 4.694935687864747, 4.71238898038469, 4.729842272904633, 4.747295565424576, 4.764748857944519, 4.782202150464463, 4.799655442984406, 4.81710873550435, 4.834562028024293, 4.852015320544236, 4.869468613064179, 4.886921905584122, 4.9043751981040655, 4.9218284906240095, 4.939281783143953, 4.956735075663896, 4.974188368183839, 4.991641660703782, 5.009094953223726, 5.026548245743669, 5.044001538263612, 5.061454830783556, 5.078908123303499, 5.096361415823442, 5.113814708343385, 5.1312680008633285, 5.148721293383272, 5.1661745859032155, 5.183627878423159, 5.201081170943102, 5.218534463463046, 5.235987755982989, 5.253441048502932, 5.270894341022875, 5.288347633542818, 5.305800926062762, 5.323254218582705, 5.340707511102648, 5.358160803622591, 5.3756140961425345, 5.393067388662478, 5.410520681182422, 5.427973973702365, 5.445427266222309, 5.462880558742252, 5.480333851262195, 5.497787143782138, 5.515240436302081, 5.532693728822024, 5.550147021341967, 5.567600313861911, 5.585053606381854, 5.602506898901798, 5.619960191421741, 5.6374134839416845, 5.654866776461628, 5.672320068981571, 5.689773361501514, 5.707226654021458, 5.724679946541401, 5.742133239061344, 5.759586531581287, 5.77703982410123, 5.794493116621174, 5.811946409141117, 5.82939970166106, 5.846852994181004, 5.8643062867009474, 5.8817595792208905, 5.899212871740834, 5.916666164260777, 5.93411945678072, 5.951572749300664, 5.969026041820607, 5.98647933434055, 6.003932626860494, 6.021385919380437, 6.03883921190038, 6.056292504420323, 6.073745796940266, 6.09119908946021, 6.1086523819801535, 6.126105674500097, 6.14355896702004, 6.161012259539983, 6.178465552059926, 6.19591884457987, 6.213372137099813, 6.230825429619757, 6.2482787221397, 6.265732014659643] ("x*y"), 3:w285) -> (0:w291:dbl[], 1:w288:dbl[])
          n188 = Merge Signals(w281, w279) -> (→"Waveform Graph":dynamicdata)
          n189 = Add(x=w285, y=w288) -> (x+y=w287:dbl[])
          n190 = call "Convert to Dynamic Data4"("Array"=w291) -> ("Dynamic Data Type"=w290:dynamicdata)  [unwired: 3 in]
          n191 = call "Convert to Dynamic Data3"("Array"=w287) -> ("Dynamic Data Type"=w293:dynamicdata)  [unwired: 3 in]
          n192 = Merge Signals(w295, w290) -> (w292:dynamicdata)
          n193 = Merge Signals(w296, w293) -> (w294:dynamicdata)
          n194 = call "Build XY Graph"("Y Input"=w292, "X Input"=w294) -> ("XY Graph"=→"XY Graph":cluster{"X":dbl[], "Y":dbl[]}[])  [unwired: 8 in, 1 out]
        }
        frame Disabled {
        }
      }
    }
  }
